vi "Get Laser State.vi"(8 "error in (no error)":errorcluster, 11 "object in":refnum<class "Laser Ethernet Cabinet.lvclass">) -> (0 "error out":errorcluster, 3 "object out":refnum<class "Laser Ethernet Cabinet.lvclass">)   [LabVIEW 2023, in "Laser Ethernet Cabinet.lvclass"]
uses:
  Laser Ethernet Cabinet.lvclass
  C:/Users/TimBerrier/Code/LabVIEW/Source/APIs/IPG/ipg_tcp/Laser_Ethernet_class/Laser_Ethernet.lvclass
  Laser Ethernet Cabinet.lvclass/Laser Ethernet Cabinet.ctl
  Laser_Ethernet_class/Laser_Ethernet.lvclass
panel:
  in  "timeout ms (25000)":i32
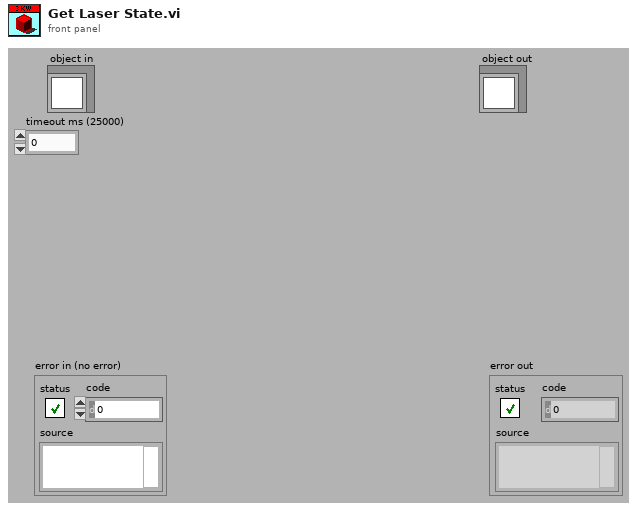
[diagram p1: front panel]
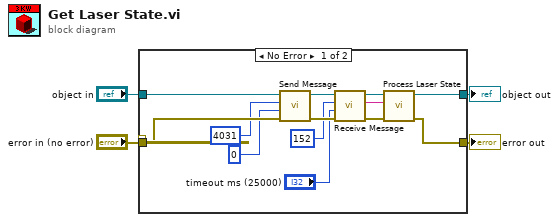
[diagram p0: block diagram]
diagram:
  n1 = case shown="No Error" "error in (no error)" {
    selector: "error in (no error)" -> [_ w18]
    tunnel: "object in" -> [w17 w19]
    tunnel: "error in (no error)" -> [w16 _]
    tunnel: [w8 w18] -> w2
    tunnel: [w9 w19] -> w1
    frame No Error {
      n2 = call "Send Message.vi"("error in (no error)"=w16, "Size of Data"=u32 0, "Command"=u16 4031, "object in"=w17) -> ("error out"=w14:errorcluster, "object out"=w15:refnum<class "Laser Ethernet Cabinet.lvclass">)  [unwired: 6 in]
      n3 = call "Receive Message.vi"("error in (no error)"=w14, "timeout ms (25000)"="timeout ms (25000)", "bytes to read"=152, "object in"=w15) -> ("error out"=w12:errorcluster, "Data"=w5:string, "object out"=w13:refnum<class "Laser Ethernet Cabinet.lvclass">)  [unwired: 5 in]
      n4 = call-dynamic "Process Laser State.vi"("error in (no error)"=w12, "Data"=w5, "object in"=w13) -> ("error out"=w8:errorcluster, "object out"=w9:refnum<class "Laser Ethernet Cabinet.lvclass">)  [unwired: 6 in]
    }
    frame Error {
    }
  }
  "error out" <- w2
  "object out" <- w1
